vi "BX.SetStringSize__LCR.vi"(8 "error in (no error)":errorcluster, 10 "String Control":refnum<vi> caption="String", 11 "State":T1={"Orientation"=0, "ActivePicture"={"image type"=0, "image depth"=0, "image"=[], "mask"=[], "colors"=[], "Rectangle"={"left"=0, "top"=0, "right"=0, "bottom"=0}}, "Pictures"={"Normal"={"image type"=0, "image depth"=0, "image"=[], "mask"=[], "colors"=[], "Rectangle"={"left"=0, "top"=0, "right"=0, "bottom"=0}}, "Hilite"={"image type"=0, "image depth"=0, "image"=[], "mask"=[], "colors"=[], "Rectangle"={"left"=0, "top"=0, "right"=0, "bottom"=0}}}, "Text"={"String"="", "Font"={"Font Name:"="", "Size"=0, "Strikeout?"=FALSE, "Italic?"=FALSE, "Underline?"=FALSE, "Outline?"=FALSE, "Shadow?"=FALSE, "Bold?"=FALSE}, "TextColor"=0}, "RunTimeSettings"={"Highlight"=FALSE, "ShowButton"=TRUE, "Behaviour"=enum."Switch when pressed", "React if disabled"=FALSE, "Nudge Button"=TRUE, "ShowButton on Hover"=FALSE, "Button Type"=enum."System"}, "Messages"=[], "Status"=0, "XControl Label"="", "Boolean Value"=FALSE} {"Status" format="%.0x"}) -> (0 "error out":errorcluster)   [LabVIEW 2011, in "BooleanXControl__LCR.xctl"]
doc: "Set the size of the string according to data inside String control"
uses:
  BooleanXControl__LCR.xctl
  Abilities/BX.State__LCR.ctl
  Controls/BX.Orientation__LCR.ctl
  <vilib>/picture/picture.llb/imagedata.ctl
  Controls/BX.RTSettings__LCR.ctl
  Controls/BX.Behaviour__LCR.ctl
  Controls/BX.ButtonType__LCR.ctl
  Controls/BX.Message__LCR.ctl
  Controls/BX.Commands__LCR.ctl
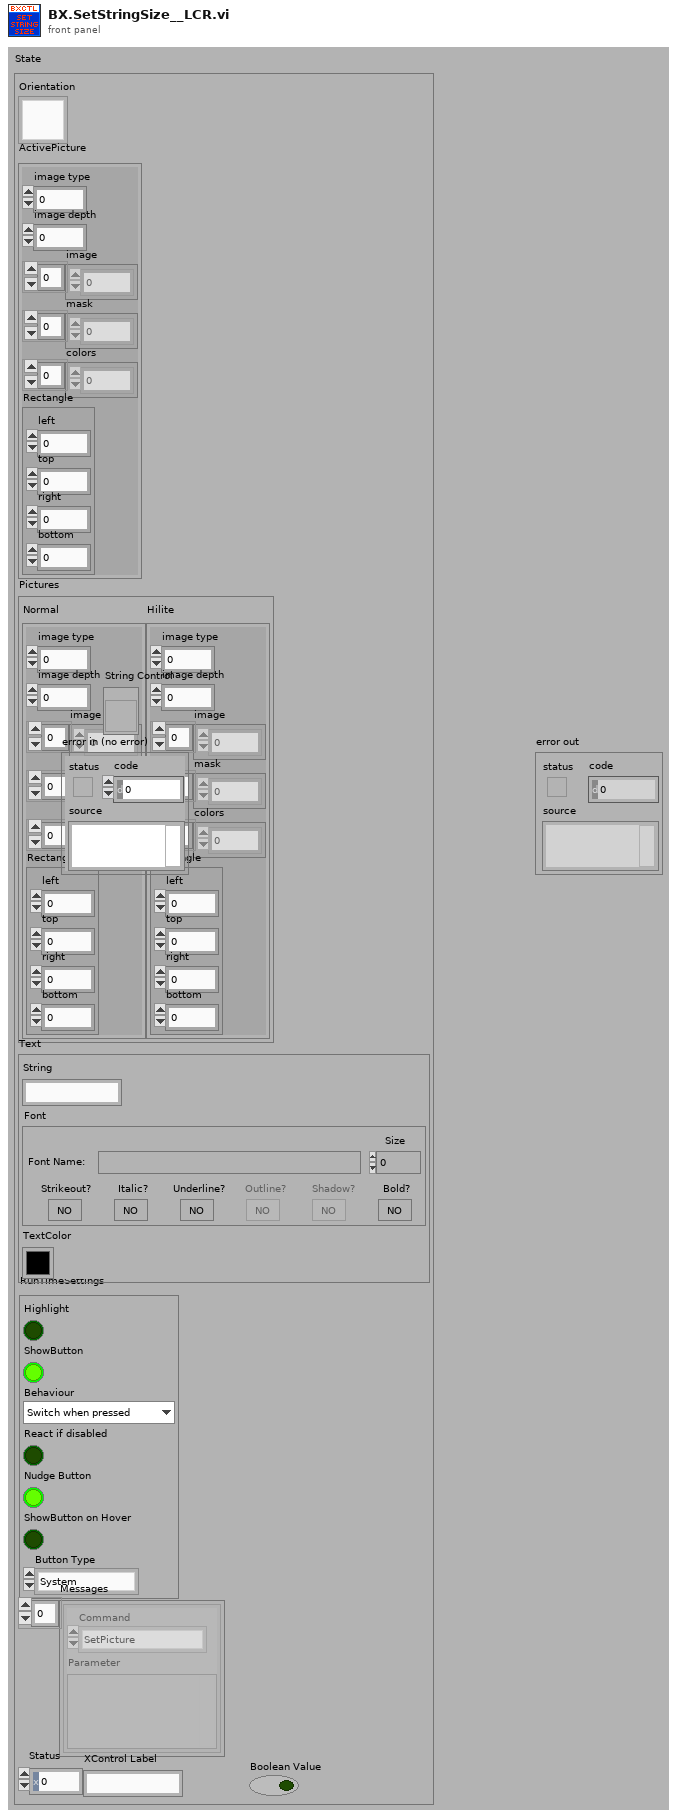
[diagram p1: front panel]
types:
  T1 = typedef "BooleanXControl__LCR.xctl/BX.State__LCR.ctl" = cluster{"Orientation":T2, "ActivePicture":T3, "Pictures":cluster{"Normal":T3, "Hilite":T3}, "Text":cluster{"String":string, "Font":cluster{"Font Name:":string, "Size":i16, "Strikeout?":bool, "Italic?":bool, "Underline?":bool, "Outline?":bool, "Shadow?":bool, "Bold?":bool}, "TextColor":u32}, "RunTimeSettings":T4, "Messages":T7[], "Status":u16, "XControl Label":string, "Boolean Value":bool}
  T2 = typedef "BooleanXControl__LCR.xctl/BX.Orientation__LCR.ctl" = u8
  T3 = typedef "imagedata.ctl" = cluster{"image type":i32, "image depth":i32, "image":u8[], "mask":u8[], "colors":u32[], "Rectangle":cluster{"left":i16, "top":i16, "right":i16, "bottom":i16}}
  T4 = typedef "BooleanXControl__LCR.xctl/BX.RTSettings__LCR.ctl" = cluster{"Highlight":bool, "ShowButton":bool, "Behaviour":T5, "React if disabled":bool, "Nudge Button":bool, "ShowButton on Hover":bool, "Button Type":T6}
  T5 = typedef "BooleanXControl__LCR.xctl/BX.Behaviour__LCR.ctl" = enum16{"Switch when pressed", "Switch when released", "Switch until released"}
  T6 = typedef "BooleanXControl__LCR.xctl/BX.ButtonType__LCR.ctl" = enum16{"System", "Modern", "Classic", "Decoration"}
  T7 = typedef "BooleanXControl__LCR.xctl/BX.Message__LCR.ctl" = cluster{"Command":T8, "Parameter":variant}
  T8 = typedef "BooleanXControl__LCR.xctl/BX.Commands__LCR.ctl" = enum16{"None", "SetPicture", "SetFont", "SetText", "SetOrientation", "Redraw", "SetTextColor", "SetRTSettings", "MultipleUpdate", "RT.Button", "RT.Hilite", "RT.Behaviour", "RT.Disabled", "ShowGUI", "RT.Nudge", "RT.Hover", "RT.ButtonType"}
  T9 = cluster{"horizontal":enum16{"left", "center", "right"}, "vertical":enum16{"top", "center", "bottom"}}
  T10 = enum16{"None", "Stacked", "Clockwise", "Counterclockwise"}
  T11 = enum16{"User-specified Font", "Application Font", "System Font", "Dialog Font"}
  T12 = cluster{"Font Name:":string, "Size":i16, "Strikeout?":bool, "Italic?":bool, "Underline?":bool, "Outline?":bool, "Shadow?":bool, "Bold?":bool}
  T13 = cluster{"left":i16, "top":i16, "right":i16, "bottom":i16}
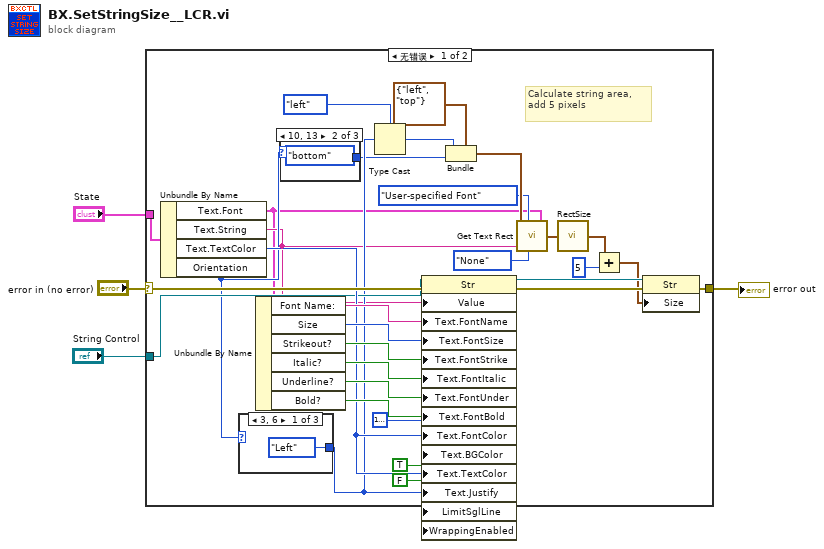
[diagram p0: block diagram]
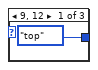
[diagram p2: hidden frame]
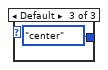
[diagram p3: hidden frame]
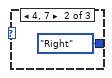
[diagram p4: hidden frame]
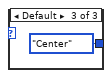
[diagram p5: hidden frame]
diagram:
  n1 = case shown="无错误" "error in (no error)" {
    selector: "error in (no error)" -> [w35 w42]
    tunnel: [w11 w42] -> w3
    tunnel: "State" -> [w15 _]
    tunnel: "String Control" -> [w26 _]
    frame No Error {
      # "Calculate string area,\nadd 5 pixels"
      n2 = Unbundle By Name(w15) -> ("Text.Font"=w13:T12, "Text.String"=w14:string, "Text.TextColor"=w28:u32, "Orientation"=w18:T2)
      n3 = case shown="3, 6" w18 {
        tunnel: [enum16{"Left", "Center", "Right"}."Left" ("Text.Justification") enum16{"Left", "Center", "Right"}."Right" ("Text.Justification") enum16{"Left", "Center", "Right"}."Center" ("Text.Justification")] -> w21
        frame 3, 6 {
        }
        frame 4, 7 {
        }
        frame Default {
        }
      }
      n4 = Unbundle By Name(w13) -> ("Font Name:"=w34:string, "Size"=w33:i16, "Strikeout?"=w32:bool, "Italic?"=w31:bool, "Underline?"=w30:bool, "Bold?"=w29:bool)
      n5 = case shown="10, 13" w18 {
        tunnel: [enum16{"top", "center", "bottom"}."top" ("vertical") enum16{"top", "center", "bottom"}."bottom" ("vertical") enum16{"top", "center", "bottom"}."center" ("vertical")] -> w17
        frame 9, 12 {
        }
        frame 10, 13 {
        }
        frame Default {
        }
      }
      n6 = Type Cast(type=enum16{"left", "center", "right"}."left" ("horizontal"), x=w21) -> (*(type *) &x=w19:enum16{"left", "center", "right"})
      n7 = property class="Str"(reference=w26, error in=w35, "Value"=w14, "Text.FontName"=w34, "Text.FontSize"=w33, "Text.FontStrike"=w32, "Text.FontItalic"=w31, "Text.FontUnder"=w30, "Text.FontBold"=w29, "Text.FontColor"=w28, "Text.BGColor"=u32 16777216, "Text.TextColor"=w28, "Text.Justify"=w21, "LimitSglLine"=TRUE ("Limit To Single Line?"), "WrappingEnabled"=FALSE ("Enable Wrapping")) -> (reference out=w10:refnum<vi>, error out=w9:errorcluster)
      n8 = Bundle(cluster=T9 {"horizontal"=enum."left", "vertical"=enum."top"} ("alignment(left, top)"), "horizontal"=w19, "vertical"=w17) -> (w22:T9)
      n9 = call <vilib>:"Get Text Rect.vi"("alignment(left, top)"=w22, "desired font(Application)"=T11."User-specified Font", "text"=w14, "text orientation"=T10."None", "[user-specified font]"=w13) -> ("rect"=w8:T13)  [unwired: 4 in]
      n10 = call <vilib>:"RectSize.vi"("rect"=w8) -> ("point"=w7:cluster{"x":i16, "y":i16})
      n11 = Add(x=w7, y=i16 5 ("Numeric")) -> (x+y=w6:cluster{"x":i16, "y":i16})
      n12 = property class="Str"(reference=w10, error in=w9, "Size"=w6) -> (error out=w11:errorcluster)  [unwired: 1 out]
    }
    frame Error {
    }
  }
  "error out" <- w3
